vi "Teleop.vi"(10 "Match Info":T1={"Autonomous Elapsed Seconds"=0.0, "TeleOp Elapsed Seconds"=0.0, "Disabled Elapsed Seconds"=0.0, "Visited Autonomous"=FALSE, "Visited TeleOp"=FALSE, "Visited Disabled"=FALSE, "Autonomous Settings"={"Autonomous Style"=enum."Independent", "VI Refnum"=refnum}}, 11 "Call Context":T2) -> ()   [LabVIEW 2017]
doc: "This VI is called for each TeleOp packet received from the DS where the robot is not disabled. It is often used to read from the joysticks and update I/O or to update setpoints for timed control loops. It should complete and return within 20 milliseconds or it may miss DS packets."
uses:
  <vilib>/Rock Robotics/WPI/DriverStation/WPI_DriverStationDerivedRobotMode.ctl
  <vilib>/Rock Robotics/WPI/DriverStation/WPI_DriverStationMatch Info.ctl
  Lift States.ctl
  Robot Global Data.vi
  Joystick Values.vi
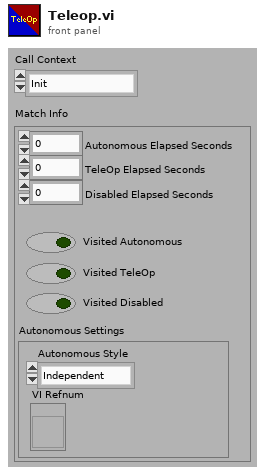
[diagram p1: front panel]
types:
  T1 = typedef "WPI_DriverStationMatch Info.ctl" = cluster{"Autonomous Elapsed Seconds":dbl, "TeleOp Elapsed Seconds":dbl, "Disabled Elapsed Seconds":dbl, "Visited Autonomous":bool, "Visited TeleOp":bool, "Visited Disabled":bool, "Autonomous Settings":cluster{"Autonomous Style":enum16{"Iterative", "Independent"}, "VI Refnum":refnum<vi>}}
  T2 = typedef "WPI_DriverStationDerivedRobotMode.ctl" = enum16{"Init", "Execute", "Stop"}
  T3 = typedef "Lift States.ctl" = enum16{"Manual", "Scale Low", "Scale Middle", "Scale High", "Rock Bottom", "Almost Down"}
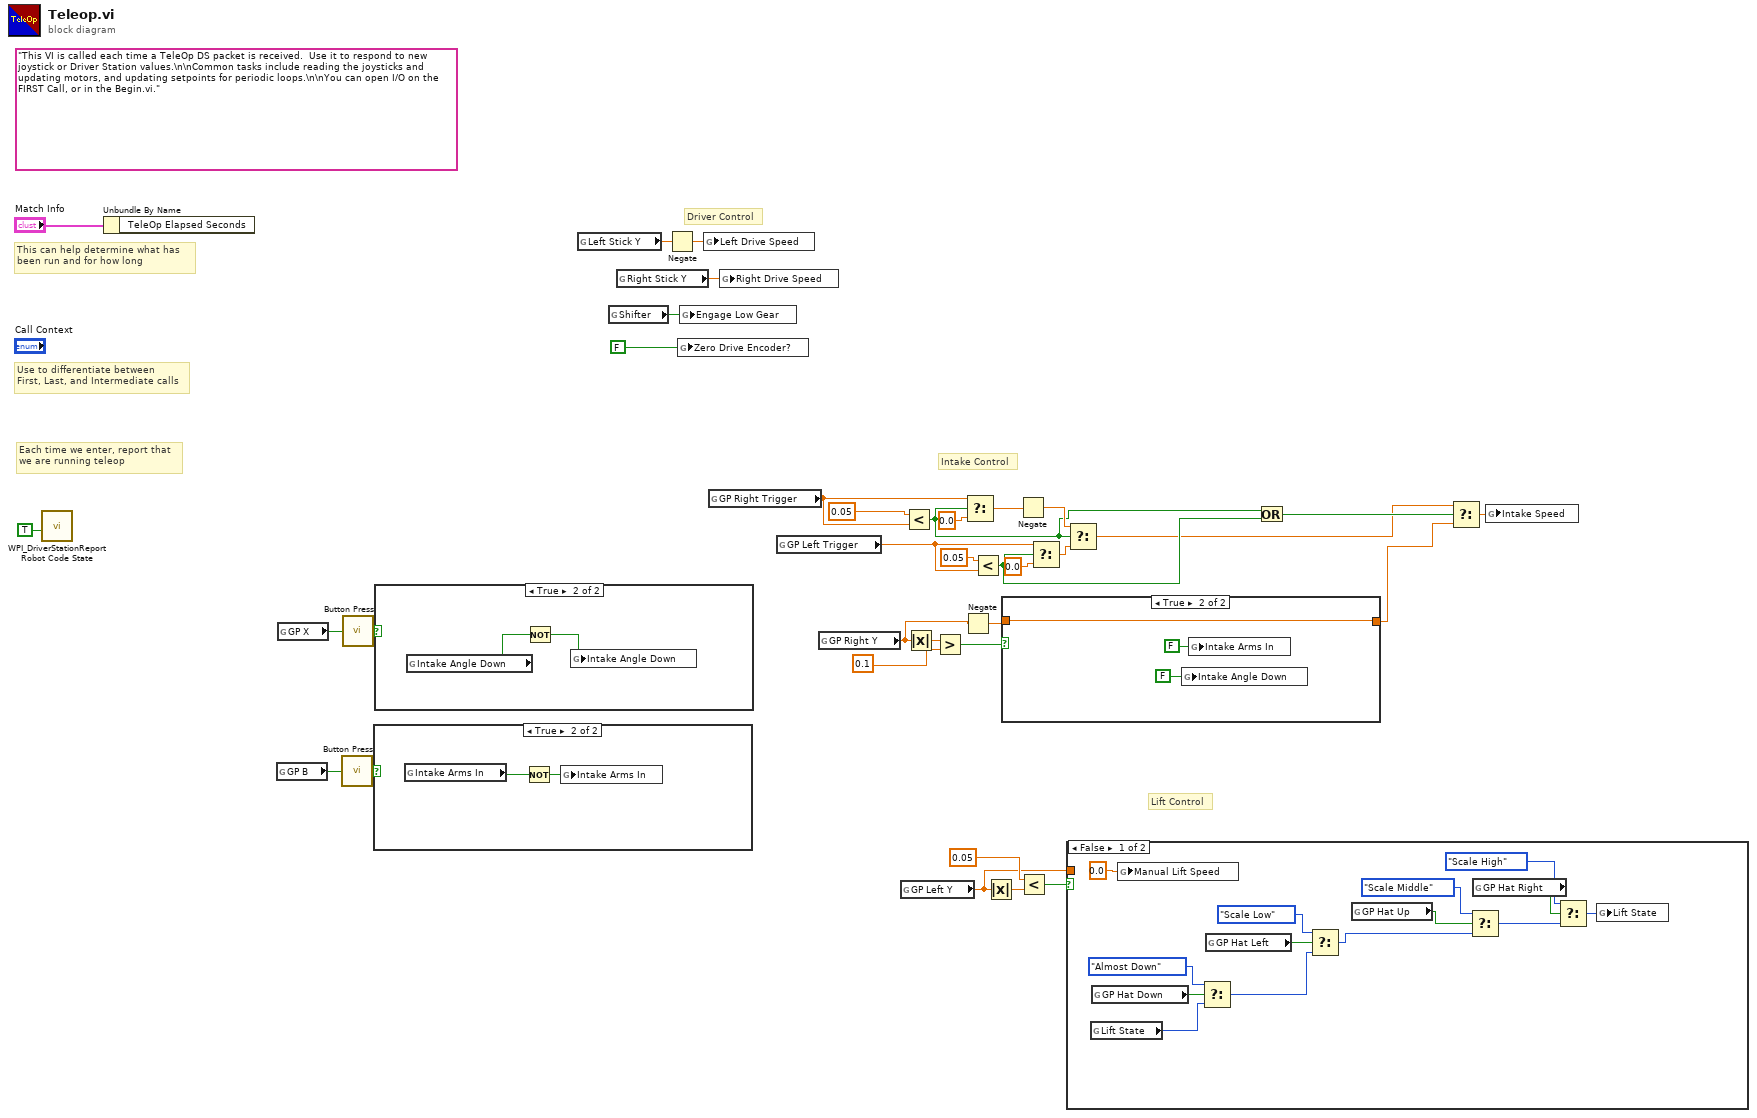
[diagram p0: block diagram]
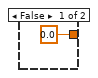
[diagram p2: hidden frame]
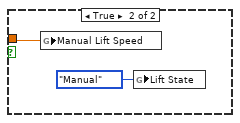
[diagram p5: hidden frame]
diagram:
  (unwired) "This VI is called each time a TeleOp DS packet is received.  Use it to respond to new joystick or Driver Station values.\n\nCommon tasks include reading the joysticks and updating motors, and updating setpoints for periodic loops.\n\nYou can open I/O on the FIRST Call, or in the Begin.vi."
  # "Driver Control"
  # "Intake Control"
  # "Lift Control"
  # "Each time we enter, report that\nwe are running teleop"
  # "Use to differentiate between\nFirst, Last, and Intermediate calls"
  # "This can help determine what has\nbeen run and for how long"
  n1 = call <vilib>:"WPI_DriverStationReport Robot Code State.vi"("TeleOp"=TRUE ("Autonomous")) -> ()  [unwired: 10 in, 1 out]
  n2 = Unbundle By Name("Match Info") -> ()  [unwired: 1 out]
  n3 = global read "Joystick Values.vi" "GP B"() -> (w17:bool)
  n4 = global read "Joystick Values.vi" "GP X"() -> (w20:bool)
  n5 = call "Button Press.vi"("Current Button"=w17) -> ("Pressed?"=w16:bool)
  n6 = call "Button Press.vi"("Current Button"=w20) -> ("Pressed?"=w19:bool)
  n7 = case shown="True" w16 {
    frame False {
    }
    frame True {
      n8 = global read "Robot Global Data.vi" "Intake Arms In"() -> (w37:bool)
      n9 = Not(x=w37) -> (.not. x?=w36:bool)
      n10 = global write "Robot Global Data.vi" "Intake Arms In"(w36) -> ()
    }
  }
  n11 = case shown="True" w19 {
    frame False {
    }
    frame True {
      n12 = global read "Robot Global Data.vi" "Intake Angle Down"() -> (w39:bool)
      n13 = Not(x=w39) -> (.not. x?=w38:bool)
      n14 = global write "Robot Global Data.vi" "Intake Angle Down"(w38) -> ()
    }
  }
  n15 = global read "Joystick Values.vi" "Left Stick Y"() -> (w5:dbl)
  n16 = global read "Joystick Values.vi" "Shifter"() -> (w3:bool)
  n17 = global read "Joystick Values.vi" "Right Stick Y"() -> (w6:dbl)
  n18 = Negate(x=w5) -> (-x=w4:dbl)
  n19 = global write "Robot Global Data.vi" "Zero Drive Encoder?"(FALSE ("Zero Drive Encoder?")) -> ()
  n20 = global write "Robot Global Data.vi" "Engage Low Gear"(w3) -> ()
  n21 = global write "Robot Global Data.vi" "Left Drive Speed"(w4) -> ()
  n22 = global read "Joystick Values.vi" "GP Right Trigger"() -> (w28:dbl)
  n23 = global write "Robot Global Data.vi" "Right Drive Speed"(w6) -> ()
  n24 = global read "Joystick Values.vi" "GP Left Trigger"() -> (w23:dbl)
  n25 = global read "Joystick Values.vi" "GP Right Y"() -> (w2:dbl)
  n26 = global read "Joystick Values.vi" "GP Left Y"() -> (w30:dbl)
  n27 = Less?(x=0.05, y=w28) -> (x < y?=w14:bool)
  n28 = Absolute Value(x=w2) -> (abs(x)=w9:dbl)
  n29 = Greater?(x=w9, y=0.1) -> (0:w8:bool)
  n30 = Negate(x=w2) -> (-x=w1:dbl)
  n31 = Select(t=w28, s=w14, f=0.0) -> (s? t:f=w26:dbl)
  n32 = Less?(x=0.05, y=w23) -> (x < y?=w15:bool)
  n33 = Absolute Value(x=w30) -> (abs(x)=w33:dbl)
  n34 = case shown="True" w8 {
    tunnel: [0.0 ("y") w41] -> w11
    tunnel: w1 -> [_ w41]
    frame False {
    }
    frame True {
      n35 = global write "Robot Global Data.vi" "Intake Angle Down"(FALSE ("Intake Arms In")) -> ()
      n36 = global write "Robot Global Data.vi" "Intake Arms In"(FALSE ("Intake Arms In")) -> ()
    }
  }
  n37 = Negate(x=w26) -> (-x=w21:dbl)
  n38 = Less?(x=0.05, y=w33) -> (x < y?=w31:bool)
  n39 = Select(t=w23, s=w15, f=0.0) -> (s? t:f=w22:dbl)
  n40 = case shown="False" w31 {
    tunnel: w30 -> [_ w58]
    frame False {
      n41 = global read "Robot Global Data.vi" "Lift State"() -> (w54:T3)
      n42 = global read "Joystick Values.vi" "GP Hat Down"() -> (w56:bool)
      n43 = global write "Robot Global Data.vi" "Manual Lift Speed"(0.0 ("Lift Speed")) -> ()
      n44 = Select(t=Lift_States."Almost Down" ("Lift State"), s=w56, f=w54) -> (s? t:f=w44:T3)
      n45 = global read "Joystick Values.vi" "GP Hat Left"() -> (w47:bool)
      n46 = Select(t=Lift_States."Scale Low" ("Lift State"), s=w47, f=w44) -> (s? t:f=w45:T3)
      n47 = global read "Joystick Values.vi" "GP Hat Up"() -> (w53:bool)
      n48 = Select(t=Lift_States."Scale Middle" ("Lift State"), s=w53, f=w45) -> (s? t:f=w51:T3)
      n49 = global read "Joystick Values.vi" "GP Hat Right"() -> (w52:bool)
      n50 = Select(t=Lift_States."Scale High" ("Lift State"), s=w52, f=w51) -> (s? t:f=w48:T3)
      n51 = global write "Robot Global Data.vi" "Lift State"(w48) -> ()
    }
    frame True {
      n52 = global write "Robot Global Data.vi" "Manual Lift Speed"(w58) -> ()
      n53 = global write "Robot Global Data.vi" "Lift State"(Lift_States."Manual" ("Lift State")) -> ()
    }
  }
  n54 = Select(t=w21, s=w14, f=w22) -> (s? t:f=w12:dbl)
  n55 = Or(x=w14, y=w15) -> (x .or. y?=w13:bool)
  n56 = Select(t=w12, s=w13, f=w11) -> (s? t:f=w10:dbl)
  n57 = global write "Robot Global Data.vi" "Intake Speed"(w10) -> ()
